vi "SetUpImageBuffer.vi"(8 "error in (no error)":errorcluster, 10 "ImageBuffers":refnum<queue>, 11 "ImagePipeline in":refnum<class "ImagePipeline.lvclass">) -> (0 "error out":errorcluster, 3 "ImagePipeline out":refnum<class "ImagePipeline.lvclass">)   [LabVIEW 2020, in "ImagePipeline.lvlib" / "ImagePipeline.lvclass"]
uses:
  ImagePipeline.lvclass
  <vilib>/vision/Image Controls.llb/IMAQ Image.ctl
  ImagePipeline.lvclass/ImagePipeline.ctl
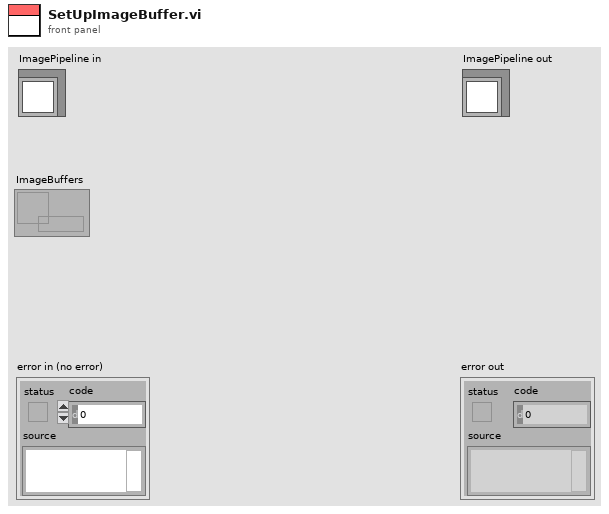
[diagram p1: front panel]
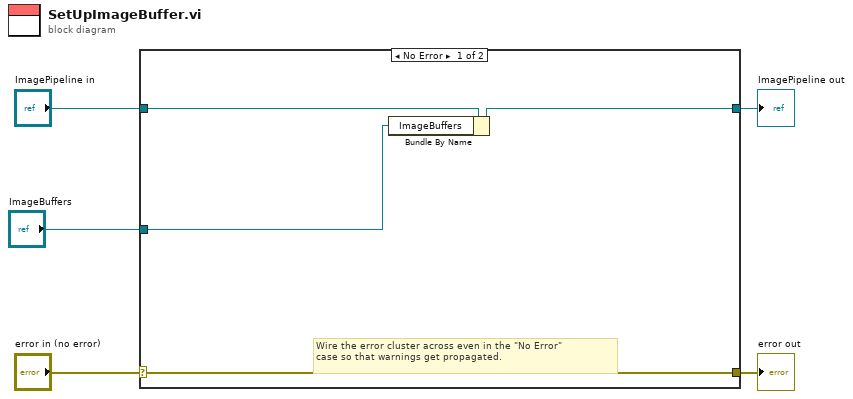
[diagram p0: block diagram]
diagram:
  n1 = case shown="No Error" "error in (no error)" {
    selector: "error in (no error)" -> [w8 w11]
    tunnel: [w8 w11] -> w4
    tunnel: [w7 w10] -> w2
    tunnel: "ImagePipeline in" -> [w9 w10]
    tunnel: "ImageBuffers" -> [w6 _]
    frame No Error {
      # "Wire the error cluster across even in the \"No Error\"\ncase so that warnings get propagated."
      n2 = Bundle By Name(cluster=w9, "ImageBuffers"=w6) -> (w7:refnum<class "ImagePipeline.lvclass">)
    }
    frame Error {
    }
  }
  "error out" <- w4
  "ImagePipeline out" <- w2
